vi "readMatFile.vi"(8 "error in (no error)":errorcluster, 9 "Skip Col Idx":i32[](array[numeric]), 10 "Skip Row Idx":i32[](array[numeric]), 11 "Path":path) -> (0 "error out":errorcluster, 3 "Matrix":dbl[][](array[numeric]))   [LabVIEW 2016]
doc: "Read the 2D matrix data from file."
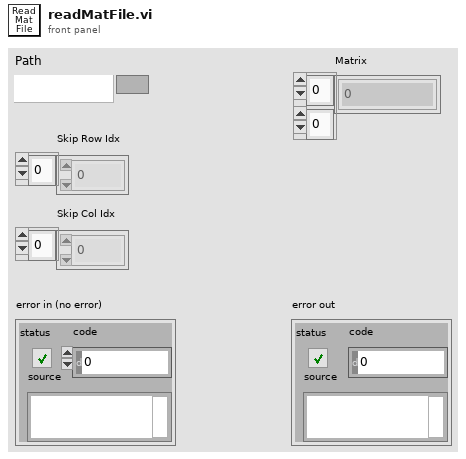
[diagram p1: front panel]
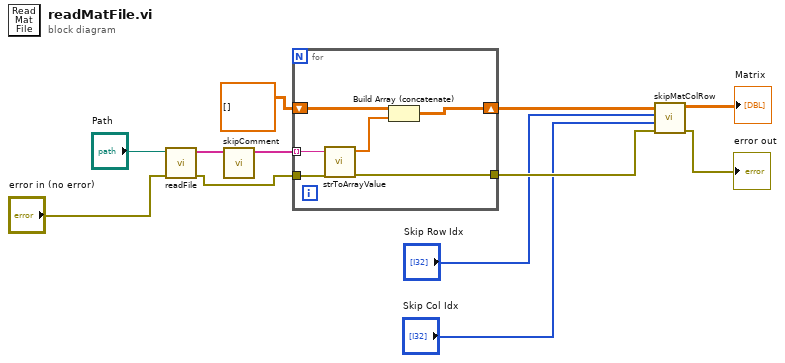
[diagram p0: block diagram]
diagram:
  n1 = call "readFile.vi"("error in (no error)"="error in (no error)", "Path"="Path") -> ("error out"=w7:errorcluster, "Array"=w12:string[])  [unwired: 8 in]
  n2 = call "skipComment.vi"("Content"=w12) -> ("Content"=w11:string[])  [unwired: 10 in]
  n3 = for {
    tunnel: w11 -> [w18] mode=indexing
    shift-right: [w15] -> w6
    shift-left: dbl[][] [] -> [w16]
    tunnel: w7 -> [w14]
    tunnel: [w13] -> w4
    n4 = call "strToArrayValue.vi"("error in (no error)"=w14, "String"=w18) -> ("error out"=w13:errorcluster, "Array"=w17:dbl[])  [unwired: 8 in]
    n5 = Build Array (concatenate)(w16, w17) -> (w15:dbl[][])
  }
  n6 = call "skipMatColRow.vi"("error in (no error)"=w4, "Skip Col Idx"="Skip Col Idx", "Skip Row Idx"="Skip Row Idx", "Matrix"=w6) -> ("error out"=→"error out":errorcluster, "Sub-Array"=→"Matrix":dbl[][])  [unwired: 6 in]
